vi "ElevatorBase_slnd.vi"(11 "ElevBasePosIn":T1=enum."Hatch") -> ()   [LabVIEW 2018]
uses:
  ElevBasePos.ctl
  <vilib>/Rock Robotics/WPI/Solenoid/Deprecated/WPI_SolenoidSetBool.vi
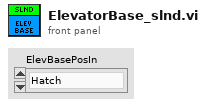
[diagram p1: front panel]
types:
  T1 = typedef "ElevBasePos.ctl" = enum16{"NoChange", "Hatch", "Unused", "Carry", "Cargo"}
  T2 = typedef "WPI_SolenoidDevRef.ctl" = cluster{"DevStatus":errorcluster, "Pneumatics Control Module":u8, "Forward Solenoid Channel":T3, "Reverse Solenoid Channel":T3}
  T3 = typedef "WPI_SolenoidChannel.ctl" = enum8{"Solenoid 0", "Solenoid 1", "Solenoid 2", "Solenoid 3", "Solenoid 4", "Solenoid 5", "Solenoid 6", "Solenoid 7", "Invalid"}
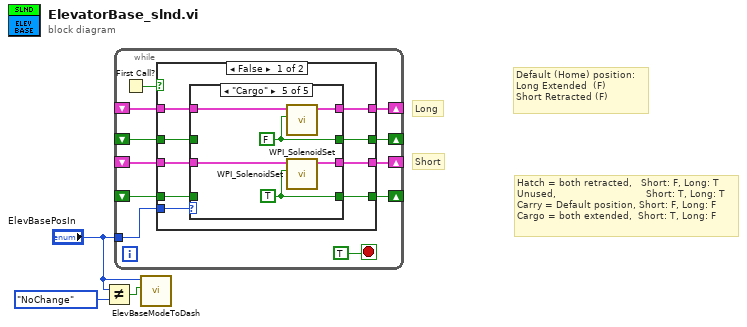
[diagram p0: block diagram]
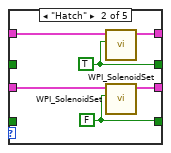
[diagram p3: hidden frame]
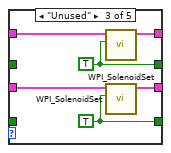
[diagram p4: hidden frame]
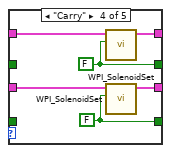
[diagram p5: hidden frame]
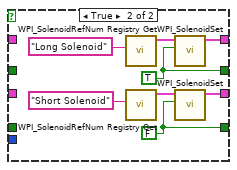
[diagram p6: hidden frame]
diagram:
  # "Default (Home) position:\nLong Extended  (F)\nShort Retracted (F)"
  # "Hatch = both retracted,   Short: F, Long: T\nUnused,                              Short: T, Long: T\nCarry = Default position, Short: F, Long: F\nCargo = both extended,  Short: T, Long: F"
  # "Short"
  # "Long"
  n1 = Not Equal?(x="ElevBasePosIn", y=ElevBasePos."NoChange" ("ElevBasePosIn 2")) -> (x != y?=w2:bool)
  n2 = while {
    shift-right: [w13] -> _
    shift-left: _ -> [w11]
    shift-right: [w12] -> _
    shift-left: _ -> [w10]
    shift-right: [w9] -> _
    shift-left: _ -> [w7]
    shift-right: [w8] -> _
    shift-left: _ -> [w6]
    tunnel: "ElevBasePosIn" -> [w4]
    stop <- TRUE stop-if-true
    n3 = First Call?() -> (First Call?: T/F=w5:bool)
    n4 = case shown="False" w5 {
      tunnel: [w23 w56] -> w13
      tunnel: [w22 w57] -> w12
      tunnel: w11 -> [w21 _]
      tunnel: w10 -> [w20 _]
      tunnel: [w18 w53] -> w9
      tunnel: [w16 w52] -> w8
      tunnel: w7 -> [w19 _]
      tunnel: w6 -> [w17 _]
      tunnel: w4 -> [w15 _]
      frame False {
        n5 = case shown="\"Cargo\"" w15 {
          tunnel: [w27 w33 w39 w45 w51] -> w23
          tunnel: [w26 w32 w38 w44 w50] -> w22
          tunnel: w21 -> [w27 w31 w37 w43 w49]
          tunnel: w20 -> [w26 w30 w36 w42 w48]
          tunnel: w19 -> [w25 _ _ _ _]
          tunnel: [w25 w28 w35 w41 w46] -> w18
          tunnel: w17 -> [w24 _ _ _ _]
          tunnel: [w24 w29 w34 w40 w47] -> w16
          frame "NoChange", Default {
          }
          frame "Hatch" {
            w29 = TRUE
            w28 = FALSE
            n6 = call-poly <vilib>:"WPI_SolenoidSet.vi"("Value"=w29, "SolenoidDevRef"=w30) -> ("SolenoidDevRef"=w32:T2)  [unwired: 8 in, 1 out]
            n7 = call-poly <vilib>:"WPI_SolenoidSet.vi"("Value"=w28, "SolenoidDevRef"=w31) -> ("SolenoidDevRef"=w33:T2)  [unwired: 8 in, 1 out]
          }
          frame "Unused" {
            w34 = TRUE
            w35 = TRUE
            n8 = call-poly <vilib>:"WPI_SolenoidSet.vi"("Value"=w34, "SolenoidDevRef"=w36) -> ("SolenoidDevRef"=w38:T2)  [unwired: 8 in, 1 out]
            n9 = call-poly <vilib>:"WPI_SolenoidSet.vi"("Value"=w35, "SolenoidDevRef"=w37) -> ("SolenoidDevRef"=w39:T2)  [unwired: 8 in, 1 out]
          }
          frame "Carry" {
            w40 = FALSE
            w41 = FALSE
            n10 = call-poly <vilib>:"WPI_SolenoidSet.vi"("Value"=w40, "SolenoidDevRef"=w42) -> ("SolenoidDevRef"=w44:T2)  [unwired: 8 in, 1 out]
            n11 = call-poly <vilib>:"WPI_SolenoidSet.vi"("Value"=w41, "SolenoidDevRef"=w43) -> ("SolenoidDevRef"=w45:T2)  [unwired: 8 in, 1 out]
          }
          frame "Cargo" {
            w47 = FALSE
            w46 = TRUE
            n12 = call-poly <vilib>:"WPI_SolenoidSet.vi"("Value"=w47, "SolenoidDevRef"=w48) -> ("SolenoidDevRef"=w50:T2)  [unwired: 8 in, 1 out]
            n13 = call-poly <vilib>:"WPI_SolenoidSet.vi"("Value"=w46, "SolenoidDevRef"=w49) -> ("SolenoidDevRef"=w51:T2)  [unwired: 8 in, 1 out]
          }
        }
      }
      frame True {
        w52 = TRUE
        w53 = FALSE
        n14 = call <vilib>:"WPI_SolenoidRefNum Registry Get.vi"("refnum name"="Long Solenoid") -> ("SolenoidDevRef"=w54:T2)  [unwired: 9 in, 1 out]
        n15 = call <vilib>:"WPI_SolenoidRefNum Registry Get.vi"("refnum name"="Short Solenoid") -> ("SolenoidDevRef"=w55:T2)  [unwired: 9 in, 1 out]
        n16 = call-poly <vilib>:"WPI_SolenoidSet.vi"("Value"=w52, "SolenoidDevRef"=w54) -> ("SolenoidDevRef"=w57:T2)  [unwired: 8 in, 1 out]
        n17 = call-poly <vilib>:"WPI_SolenoidSet.vi"("Value"=w53, "SolenoidDevRef"=w55) -> ("SolenoidDevRef"=w56:T2)  [unwired: 8 in, 1 out]
      }
    }
  }
  n18 = call "ElevBaseModeToDash.vi"("Update?"=w2, "ElevBasePosIn"="ElevBasePosIn") -> ()  [unwired: 9 in, 1 out]
